vi "Set Channel Class.vi"(8 "error in":errorcluster, 11 "analog input Arms mode in":refnum<class "Analog Input Arms Mode.lvclass">) -> (0 "error out":errorcluster, 3 "analog input Arms mode out":refnum<class "Analog Input Arms Mode.lvclass">)   [LabVIEW 2020, in "Scan Engine Scripting.lvlib" / "Analog Input Arms Mode.lvclass"]
uses:
  Analog Input Arms Mode.lvclass
  Channel Classes/AI Arms Channel/AI Arms Channel.lvclass
  C:/jenkins/workspace/ercat-custom-device_release_20.4/Custom Device Source/Scripting/Modules/Channel Classes/AI Channel/AI Channel.lvclass
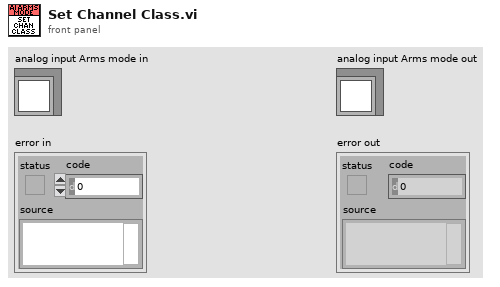
[diagram p1: front panel]
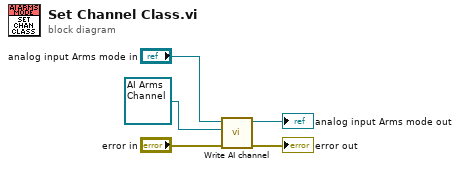
[diagram p0: block diagram]
diagram:
  n1 = call-dynamic "Write AI channel.vi"("error in"="error in", "analog input mode channel"=refnum<class "AI Arms Channel.lvclass"> refnum ("Scan Engine Scripting.lvlib:AI Arms Channel.lvclass"), "analog input mode in"="analog input Arms mode in") -> ("error out"=→"error out":errorcluster, "analog input mode out"=→"analog input Arms mode out":refnum<class "Analog Input Arms Mode.lvclass">)  [unwired: 7 in]
